vi "Match Sessions with Pins.vi"(9 "pin array":string[](array[string]), 11 "Sessions Info In":T1[](array[typedef])) -> (3 "Sessions Info Out":T1[](array[typedef]))   [LabVIEW 2020, in "MeasurementLink Session Management.lvlib" / "Session Reservation.lvclass"]
uses:
  Session Reservation.lvclass
  Session Reservation.lvclass/Session Reservation.ctl
  MeasurementLink Session Management Client/RPC Messages/ni_measurementlink_sessionmanagement_v1_ChannelMapping.ctl
  MeasurementLink Session Management Client/MeasurementLink Session Management Client.lvlib
  MeasurementLink Session Management Client/RPC Messages/nidevice_grpc_Session.ctl
  MeasurementLink Session Management Client/RPC Messages/ni_measurementlink_sessionmanagement_v1_SessionInformation.ctl
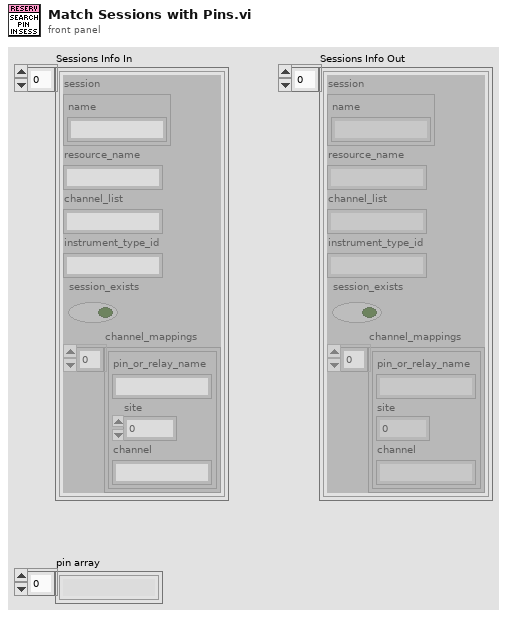
[diagram p1: front panel]
types:
  T1 = typedef "MeasurementLink Session Management Client.lvlib/ni_measurementlink_sessionmanagement_v1_SessionInformation.ctl" = cluster{"session":T2, "resource_name":string, "channel_list":string, "instrument_type_id":string, "session_exists":bool, "channel_mappings":T3[]}
  T2 = typedef "MeasurementLink Session Management Client.lvlib/nidevice_grpc_Session.ctl" = cluster{"name":string}
  T3 = typedef "MeasurementLink Session Management Client.lvlib/ni_measurementlink_sessionmanagement_v1_ChannelMapping.ctl" = cluster{"pin_or_relay_name":string, "site":i32, "channel":string}
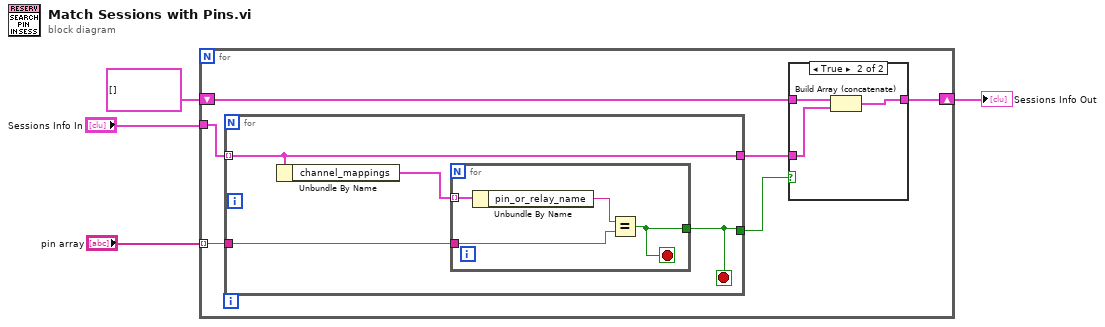
[diagram p0: block diagram]
diagram:
  n1 = for {
    tunnel: "Sessions Info In" -> [w10]
    tunnel: "pin array" -> [w9] mode=indexing
    shift-right: [w5] -> w1
    shift-left: T1[] [] ("sessions info") -> [w6]
    n2 = for {
      tunnel: w10 -> [w15] mode=indexing
      tunnel: w9 -> [w17]
      tunnel: [w15] -> w7
      tunnel: [w16] -> w8
      stop <- w16 stop-if-true
      n3 = Unbundle By Name(w15) -> ("channel_mappings"=w18:T3[])
      n4 = for {
        tunnel: w18 -> [w22] mode=indexing
        tunnel: w17 -> [w20]
        tunnel: [w19] -> w16
        stop <- w19 stop-if-true
        n5 = Unbundle By Name(w22) -> ("pin_or_relay_name"=w21:string)
        n6 = Equal?(x=w21, y=w20) -> (x = y?=w19:bool)
      }
    }
    n7 = case shown="True" w8 {
      tunnel: w7 -> [_ w14]
      tunnel: w6 -> [w11 w13]
      tunnel: [w11 w12] -> w5
      frame False {
      }
      frame True {
        n8 = Build Array (concatenate)(w13, w14) -> (w12:T1[])
      }
    }
  }
  "Sessions Info Out" <- w1
